vi "Create Circle Cluster.vi"(6 "B":dbl, 9 "HorCenter":u16, 10 "VerCenter":u32, 11 "A":dbl) -> (3 "Bounding Rectangle":T1)   [LabVIEW 2015]
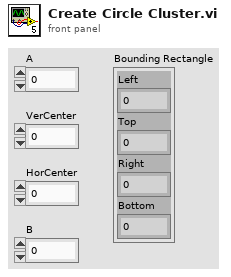
[diagram p1: front panel]
types:
  T1 = cluster{"Left":i32, "Top":i32, "Right":i32, "Bottom":i32}
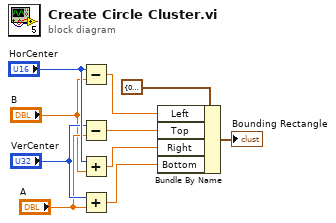
[diagram p0: block diagram]
diagram:
  n1 = Subtract(x="HorCenter", y="B") -> (x-y=w2:dbl)
  n2 = Subtract(x="VerCenter", y="A") -> (x-y=w4:dbl)
  n3 = Add(x="HorCenter", y="B") -> (x+y=w3:dbl)
  n4 = Add(x="VerCenter", y="A") -> (x+y=w5:dbl)
  n5 = Bundle By Name(cluster=T1 {"Left"=0, "Top"=0, "Right"=0, "Bottom"=0} ("Bounding Rectangle"), "Left"=w2, "Top"=w4, "Right"=w3, "Bottom"=w5) -> (→"Bounding Rectangle":T1)
